vi "set magnet read detector and hall probe.vi"(6 "Field settle time (400 msec)":dbl=400.0, 8 "error in (no error)":errorcluster, 9 "Magnet voltage":dbl, 10 "Input task":refnum<k21>, 11 "Output task":refnum<k21>) -> (0 "error out":errorcluster, 1 "Data":dbl[](array[numeric]), 2 "Input task":refnum<k21>, 3 "Output task":refnum<k21>)   [LabVIEW 2014]
uses:
  <vilib>/GPower/Math/Library/Stat/Mean/MeanDBL.vi
  <vilib>/DAQmx/write.llb/DAQmx Write (Analog DBL 1Chan 1Samp).vi
  <vilib>/DAQmx/read.llb/DAQmx Read (Analog 2D DBL NChan NSamp).vi
  <vilib>/GPower/Math/GPMath.lvlib
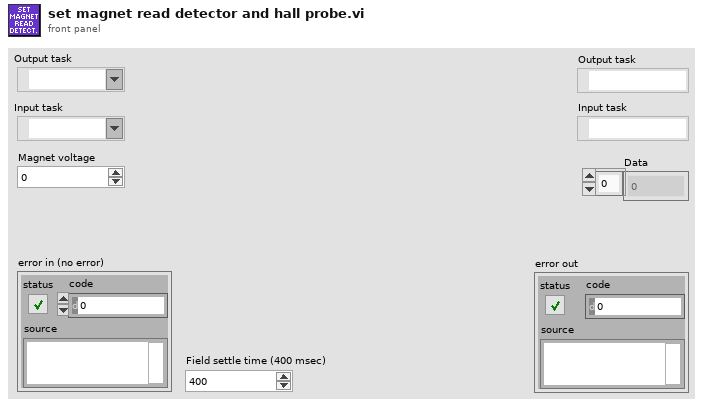
[diagram p1: front panel]
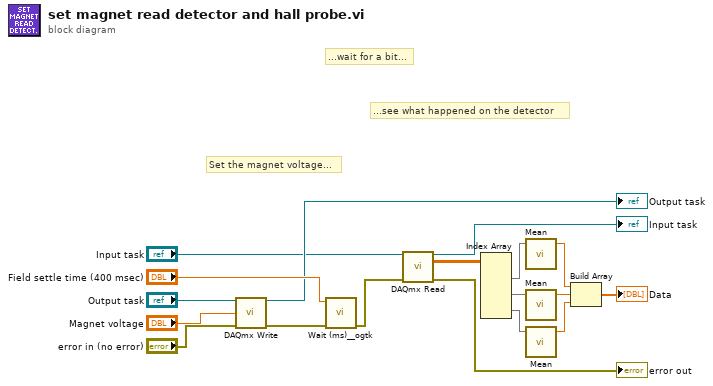
[diagram p0: block diagram]
diagram:
  # "...see what happened on the detector"
  # "...wait for a bit..."
  # "Set the magnet voltage..."
  n1 = call-poly <vilib>:"DAQmx Write.vi"("task/channels in"="Output task", "data"="Magnet voltage", "error in"="error in (no error)") -> ("task out"=→"Output task":refnum<k21>, "error out"=w16:errorcluster)  [unwired: 10 in, 1 out]
  n2 = call <userlib>:"Wait (ms)__ogtk.vi"("error in (no error)"=w16, "milliseconds to wait"="Field settle time (400 msec)") -> ("error out"=w18:errorcluster)  [unwired: 8 in, 1 out]
  n3 = call-poly <vilib>:"DAQmx Read.vi"("task/channels in"="Input task", "error in"=w18) -> ("task out"=→"Input task":refnum<k21>, "data"=w8:dbl[][], "error out"=→"error out":errorcluster)  [unwired: 11 in]
  n4 = Index Array(array=w8) -> (element #1=w7:dbl[], element #2=w6:dbl[], element #3=w5:dbl[])  [unwired: 6 in]
  n5 = call-poly <vilib>:"Mean.vi"("X"=w7) -> ("Mean"=w4:dbl)  [unwired: 4 in]
  n6 = call-poly <vilib>:"Mean.vi"("X"=w6) -> ("Mean"=w3:dbl)  [unwired: 4 in]
  n7 = call-poly <vilib>:"Mean.vi"("X"=w5) -> ("Mean"=w2:dbl)  [unwired: 4 in]
  n8 = Build Array(w4, w3, w2) -> (→"Data":dbl[])
